vi "Sequence Read.vi"(8 "error in (no error)":errorcluster, 11 "MSX-E3711 in":refnum<class "MSX-E3711.lvclass">) -> (0 "error out":errorcluster, 1 "Control Data":T1, 2 "Acquisition Data":T2[](array[typedef]), 3 "MSX-E3711 out":refnum<class "MSX-E3711.lvclass">)   [LabVIEW 2014, in "MSX-E3711.lvlib" / "MSX-E3711.lvclass"]
uses:
  MSX-E3711.lvclass
  DriverMasterSync/build/DriverMasterSync.lvlibp/APIs/Data Queue/Acquisition Data 1 Sample Cluster.ctl
  DriverMasterSync/build/DriverMasterSync.lvlibp/APIs/Data Queue/Control Data Cluster.ctl
  MSX-E3711.lvclass/MSX-E3711.ctl
  DriverMasterSync/build/DriverMasterSync.lvlibp/Modules/HAL/DriverMasterSync/DriverMasterSyncClass/DriverMasterSync.lvclass
  API/MSX-E3711_dll.lvlib
  DriverMasterSync/build/DriverMasterSync.lvlibp/APIs/Data Queue/WINFAS 2 Data Queue.lvlib
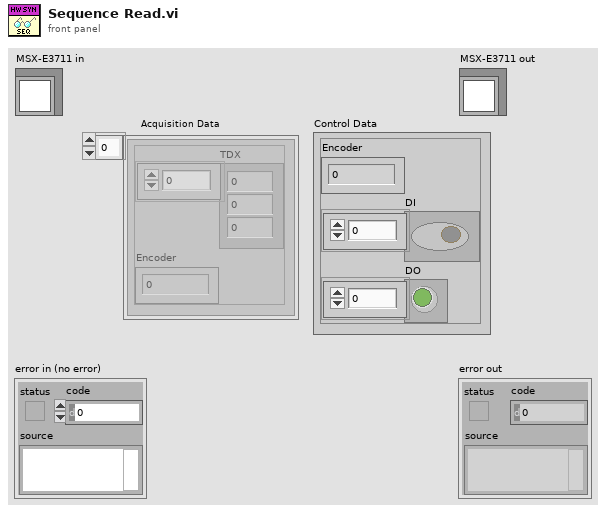
[diagram p1: front panel]
types:
  T1 = typedef "DriverMasterSync.lvlibp/WINFAS 2 Data Queue.lvlib/Control Data Cluster.ctl" = cluster{"Encoder":sgl, "DI":bool[], "DO":bool[]}
  T2 = typedef "DriverMasterSync.lvlibp/WINFAS 2 Data Queue.lvlib/Acquisition Data 1 Sample Cluster.ctl" = cluster{"TDX":sgl[], "Encoder":sgl}
  T3 = typedef "DriverMasterSync.lvlibp/HAL Config Data.ctl" = cluster{"HWSync Index":u32, "Driver Name":string, "Channel Mask":u64}
  T4 = typedef "MSX-E3711_dll.lvlib/Connection Data.ctl" = cluster{"MX371x refnum":refnum<k24>, "IP":string, "Connection ID ":refnum<k5>, "MXCommon refnum":refnum<k24>}
  T5 = typedef "MSX-E3711_dll.lvlib/Config Data.ctl" = cluster{"Auto Refresh":cluster{"Average Mode":u64, "Average Value":u64, "Trigger Mask":u64, "Trigger Mode":u64, "Hardware Trigger Edge":u64, "Hardware Trigger Count":u64, "By Trigger Nbr Of Seq To Acquire":u64, "Time stamp":bool, "Analog Output(mm)":bool, "Invert value":bool, "Temperature value":bool, "Incremental counter value":bool, "Diff. mode":bool}, "Gain":sgl[], "Offset":sgl[], "Index":u64, "Range":sgl, "Sequence":cluster{"Nbr Of Sequence":u64, "Nbr Max Sequence To Transfer":u64, "Delay Mode":u64, "Delay Time Unit":u64, "Delay Value":u64, "Trigger Mask":u64, "Trigger Mode":u64, "Hardware Trigger Edge":u64, "Hardware Trigger Count":u64, "By Trigger Nbr Of Seq To Acquire":u64, "Time stamp":bool, "Sequence counter information":bool, "Analog Output(mm)":bool, "Invert value":bool, "Temperature value":bool, "Incremental counter value":bool, "Diff. mode":bool}, "Enable DIO":bool, "IncCounter":cluster{"CounterMode":string, "CounterOptionDIRECT  ":bool, "CounterOptionOthers":bool, "CounterClear ":bool, "Cantidad de Pulsos":sgl, "Reducción":sgl}, "IncTemperature":cluster{"ConnectedTempSensor":string, "ConvertMode":string, "InitGainSelection":string, "FrequencySelection":string, "PowerSaveMode":bool, "GainSelection":string, "RefValue":dbl}}
  T6 = typedef "MSX-E3711_dll.lvlib/Adquisition Data.ctl" = cluster{"Adq. Sequence":cluster{"Adquisition Value":u32[][], "Counter Value":u32[], "TSs - TSu - NAS":u64[][], "Status IO Port":bool[]}, "Adq. Auto Refresh":cluster{"Adquisition Value":u64[], "Status IO Port":bool[], "Counter value":u32}}
  T7 = cluster{"Adquisition Value":u32[][], "Counter Value":u32[], "TSs - TSu - NAS":u64[][], "Status IO Port":bool[]}
  T8 = typedef "DriverMasterSync.lvlibp/WINFAS 2 Data Queue.lvlib/Acquisition Data Cluster.ctl" = T2[]
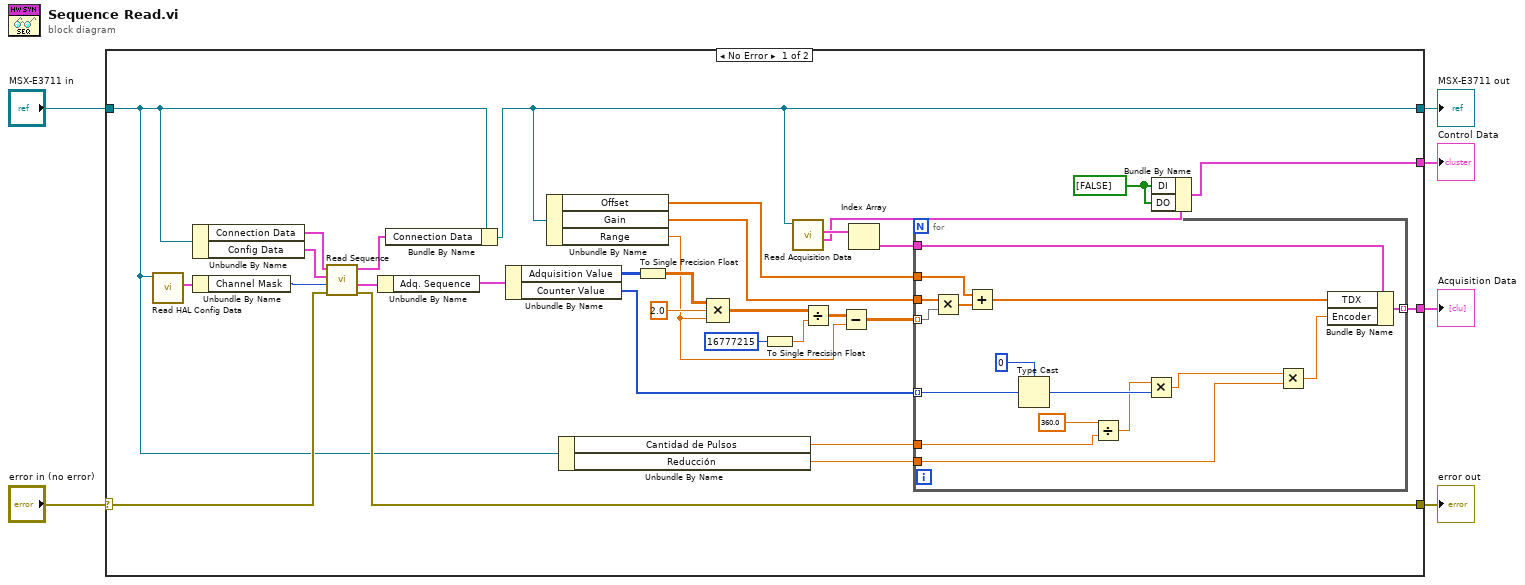
[diagram p0: block diagram]
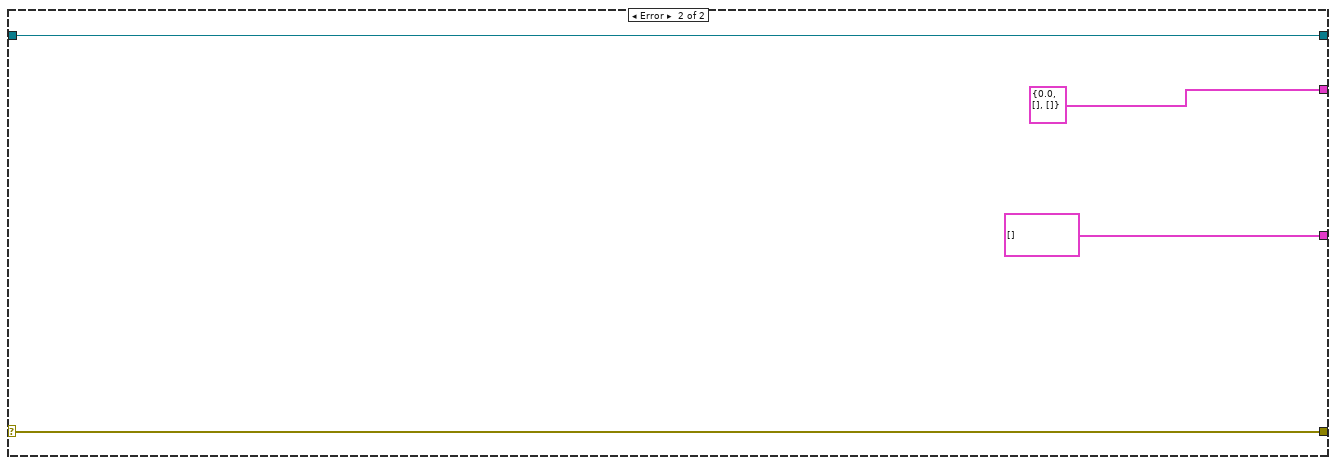
[diagram p2: hidden frame]
diagram:
  n1 = case shown="No Error" "error in (no error)" {
    selector: "error in (no error)" -> [w18 w57]
    tunnel: [w17 w57] -> w5
    tunnel: [w22 w56] -> w3
    tunnel: "MSX-E3711 in" -> [w13 w56]
    tunnel: [w16 T2[] []] -> w2
    tunnel: [w9 T1 {"Encoder"=0.0, "DI"=[], "DO"=[]} ("Control Data")] -> w1
    frame No Error {
      w8 = bool[] [FALSE] ("DI")
      n2 = call "Read HAL Config Data.vi"("DriverMasterSync in"=w13) -> ("HAL Config Data"=w24:T3)  [unwired: 8 in, 2 out]
      n3 = Unbundle By Name(w13) -> ("Connection Data"=w21:T4, "Config Data"=w20:T5)
      n4 = Unbundle By Name(w24) -> ("Channel Mask"=w19:u64)
      n5 = call "Read Sequence.vi"("error in (no error)"=w18, "Channel Mask"=w19, "Config Data"=w20, "Connection Data In"=w21) -> ("error out"=w17:errorcluster, "Adquisition Data Out"=w14:T6, "Connection Data Out"=w15:T4)  [unwired: 5 in]
      n6 = Unbundle By Name(w14) -> ("Adq. Sequence"=w37:T7)
      n7 = Bundle By Name(cluster=w13, "Connection Data"=w15) -> (w22:refnum<class "MSX-E3711.lvclass">)
      n8 = Unbundle By Name(w37) -> ("Adquisition Value"=w29:u32[][], "Counter Value"=w7:u32[])
      n9 = Unbundle By Name(w22) -> ("Offset"=w34:sgl[], "Gain"=w35:sgl[], "Range"=w25:sgl)
      n10 = Unbundle By Name(w13) -> ("Cantidad de Pulsos"=w11:sgl, "Reducción"=w12:sgl)
      n11 = To Single Precision Float(number=w29) -> (single precision float=w28:sgl[][])
      n12 = Compound Arithmetic op=MULTIPLY(w28, sgl 2.0 ("x"), w25) -> (w31:sgl[][])
      n13 = To Single Precision Float(number=u64 16777215 ("x")) -> (single precision float=w27:sgl)
      n14 = call "Read Acquisition Data.vi"("DriverMasterSync in"=w22) -> ("Control Data"=w10:T1, "Acquisition Data"=w23:T8)  [unwired: 7 in, 2 out]
      n15 = Divide(x=w31, y=w27) -> (x/y=w32:sgl[][])
      n16 = Subtract(x=w32, y=w25) -> (x-y=w30:sgl[][])
      n17 = Index Array(array=w23) -> (element=w36:T2)  [unwired: 1 in]
      n18 = for {
        tunnel: w36 -> [w53]
        tunnel: w30 -> [w51] mode=indexing
        tunnel: w35 -> [w50]
        tunnel: w34 -> [w49]
        tunnel: [w47] -> w16 mode=indexing
        tunnel: w12 -> [w45]
        tunnel: w11 -> [w40]
        tunnel: w7 -> [w43] mode=indexing
        n19 = Multiply(x=w50, y=w51) -> (x*y=w52:sgl[])
        n20 = Add(x=w49, y=w52) -> (x+y=w48:sgl[])
        n21 = Type Cast(type=0, x=w43) -> (*(type *) &x=w42:i32)
        n22 = Divide(x=sgl 360.0 ("y"), y=w40) -> (x/y=w39:sgl)
        n23 = Multiply(x=w39, y=w42) -> (x*y=w38:sgl)
        n24 = Multiply(x=w38, y=w45) -> (x*y=w46:sgl)
        n25 = Bundle By Name(cluster=w53, "TDX"=w48, "Encoder"=w46) -> (w47:T2)
      }
      n26 = Bundle By Name(cluster=w10, "DI"=w8, "DO"=w8) -> (w9:T1)
    }
    frame Error {
    }
  }
  "error out" <- w5
  "MSX-E3711 out" <- w3
  "Acquisition Data" <- w2
  "Control Data" <- w1
